vi "svc_Get Array Subset (Index).vi"(8 "error in (no error)":errorcluster, 9 "length (-1 = all)":i32=-1 min=-1 step=1, 10 "start index (0)":i32 step=1, 11 "Y":dbl[](array[numeric])) -> (0 "error out":errorcluster, 1 "actual length":i32, 2 "actual start index":i32, 3 "Y subset":dbl[](array[numeric]), 4 "end reached":bool)   [LabVIEW 2017]
doc: "Returns a portion of the waveform of the <B>start index</B> and <B>length</B> values. When you wire a waveform to this VI, the waveform automatically resizes to display <B>start index</B> inputs for the waveform."
uses:
  <vilib>/addons/_NISVFA/_Shared subVIs/Common/svc_Conditional Merge Error.vi
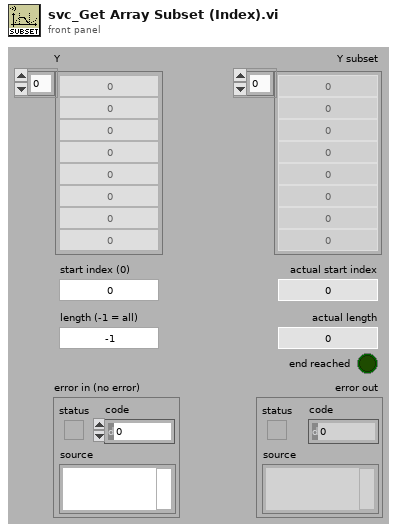
[diagram p1: front panel]
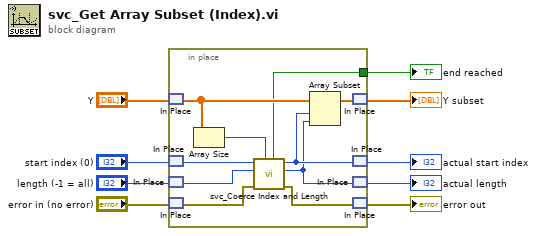
[diagram p0: block diagram]
diagram:
  n1 = in-place {
    in-place-border: [w13] -> w3
    n2 = in-place-match #1("Y") -> (w19:dbl[])
    n3 = in-place-match #2("start index (0)") -> (w14:i32)
    n4 = in-place-match #3("length (-1 = all)") -> (w15:i32)
    n5 = in-place-match #4("error in (no error)") -> (w11:errorcluster)
    n6 = Array Size(array=w19) -> (size(s)=w16:i32)
    n7 = call <vilib>:"svc_Coerce Index and Length.vi"("input length"=w16, "error in (no error)"=w11, "subset length (-1 = all)"=w15, "subset start index (0)"=w14) -> ("error out"=w10:errorcluster, "actual subset length"=w12:i32, "actual start index"=w17:i32, "end reached"=w13:bool)  [unwired: 4 in]
    n8 = Array Subset(array=w19, index=w17, length=w12) -> (w18:dbl[])
    n9 = in-place-match #1(w18) -> (→"Y subset":dbl[])
    n10 = in-place-match #2(w17) -> (→"actual start index":i32)
    n11 = in-place-match #3(w12) -> (→"actual length":i32)
    n12 = in-place-match #4(w10) -> (→"error out":errorcluster)
  }
  "end reached" <- w3
